vi "Manipulate outputs.vi"(1 "ON for":dbl, 4 "data value reference in":refnum<data-value>, 7 "Output pins":T1, 8 "Last on":timestamp, 9 "Delay":dbl, 10 "Threshold":dbl, 11 "Data":dbl) -> (0 "Time Output":timestamp, 2 "LED value":dbl, 3 "Fan value":dbl, 5 "data value reference out":refnum<data-value>)   [LabVIEW 2020]
uses:
  <vilib>/DAQmx/write.llb/DAQmx Write (Analog DBL 1Chan 1Samp).vi
  Global variable.vi
  <vilib>/DAQmx/miscellaneous.llb/DAQmx Fill In Error Info.vi
panel:
  in  "Decay speed":dbl=1.0
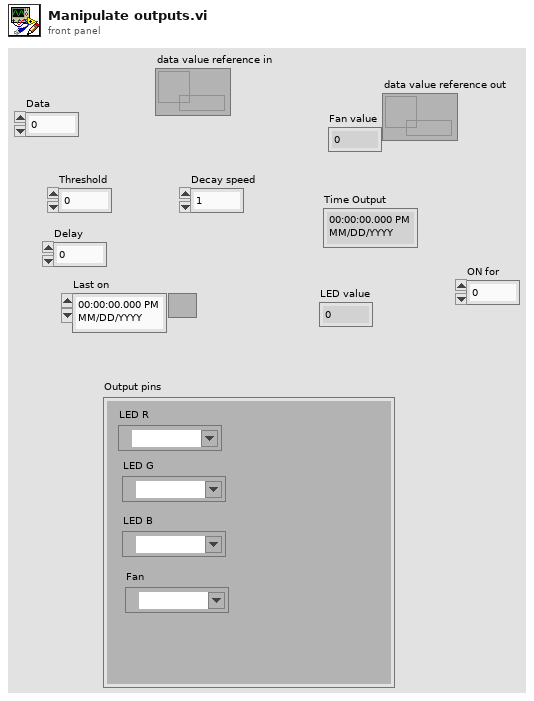
[diagram p1: front panel]
types:
  T1 = cluster{"LED R":tag, "LED G":tag, "LED B":tag, "Fan":tag}
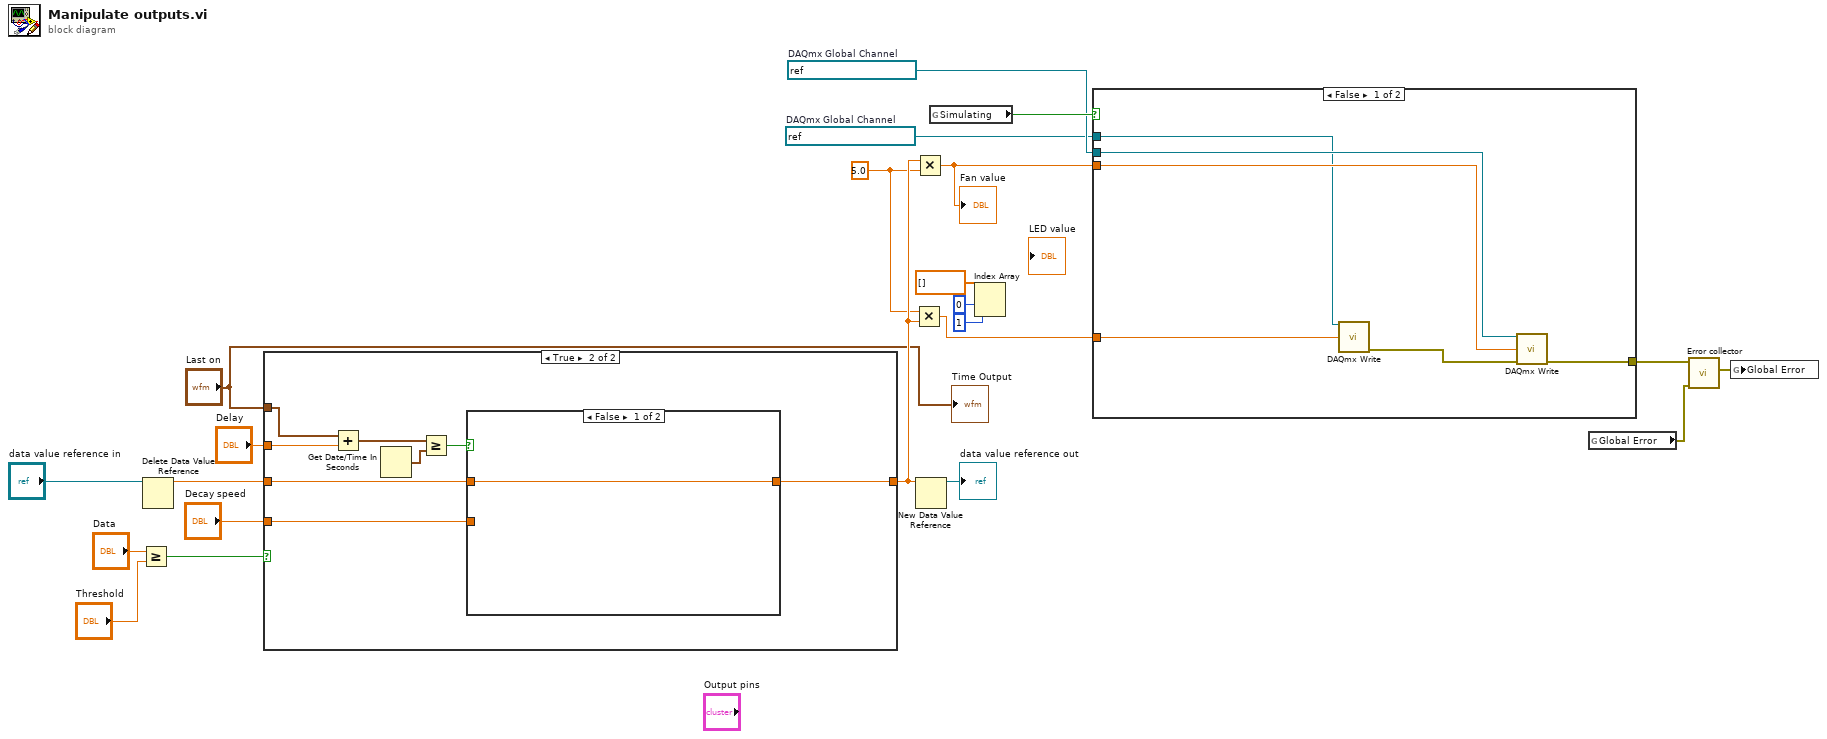
[diagram p0: block diagram]
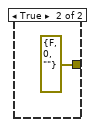
[diagram p2: hidden frame]
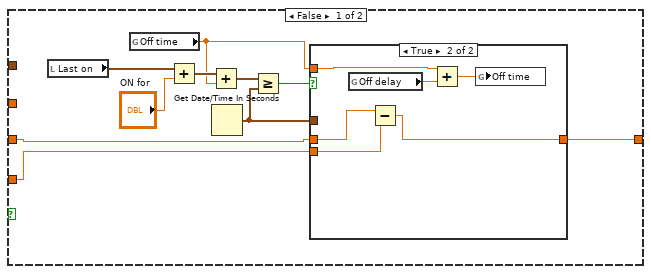
[diagram p3: hidden frame]
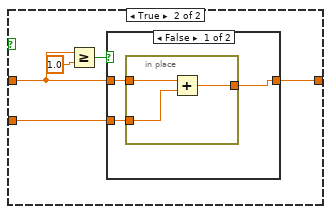
[diagram p5: hidden frame]
diagram:
  w6 = refnum<k21> "LEDOutputChannel"  # DAQmx Global Channel
  w7 = refnum<k21> "FanOutputChannel"  # DAQmx Global Channel
  w5 = 5.0
  n1 = Greater Or Equal?(x="Data", y="Threshold") -> (x >= y?=w20:bool)
  n2 = Delete Data Value Reference(data value reference="data value reference in") -> (data value=w16:dbl)  [unwired: 1 in, 1 out]
  n3 = case shown="True" w20 {
    tunnel: "Delay" -> [_ w47]
    tunnel: w16 -> [w28 w43]
    tunnel: "Decay speed" -> [w29 w42]
    tunnel: [w27 w41] -> w14
    tunnel: "Last on" -> [_ w40]
    frame False {
      n4 = local read "Last on"() -> (w31:timestamp)
      n5 = global read "Global variable.vi" "Off time"() -> (w23:dbl)
      n6 = Add(x=w31, y="ON for") -> (x+y=w24:timestamp)
      n7 = Add(x=w24, y=w23) -> (x+y=w25:timestamp)
      n8 = Get Date/Time In Seconds() -> (seconds since 1Jan1904=w26:timestamp)
      n9 = Greater Or Equal?(x=w25, y=w26) -> (x >= y?=w30:bool)
      n10 = case shown="True" w30 {
        tunnel: w29 -> [_ w39]
        tunnel: w28 -> [w33 w38]
        tunnel: [w33 w37] -> w27
        tunnel: w26 -> [_ _]
        tunnel: w23 -> [_ w35]
        frame False {
        }
        frame True {
          n11 = global read "Global variable.vi" "Off delay"() -> (w34:dbl)
          n12 = Subtract(x=w38, y=w39) -> (x-y=w37:dbl)
          n13 = Add(x=w35, y=w34) -> (x+y=w36:dbl)
          n14 = global write "Global variable.vi" "Off time"(w36) -> ()
        }
      }
    }
    frame True {
      n15 = Add(x=w40, y=w47) -> (x+y=w46:timestamp)
      n16 = Get Date/Time In Seconds() -> (seconds since 1Jan1904=w45:timestamp)
      n17 = Greater Or Equal?(x=w46, y=w45) -> (x >= y?=w44:bool)
      n18 = case shown="False" w44 {
        tunnel: w43 -> [w48 w51]
        tunnel: w42 -> [_ w50]
        tunnel: [w48 w49] -> w41
        frame False {
        }
        frame True {
          n19 = Greater Or Equal?(x=w51, y=1.0) -> (x >= y?=w52:bool)
          n20 = case shown="False" w52 {
            tunnel: w51 -> [w56 w60]
            tunnel: w50 -> [w55 _]
            tunnel: [w54 w60] -> w49
            frame False {
              n21 = in-place {
                in-place-border: w56 -> [w59]
                in-place-border: w55 -> [w58]
                in-place-border: [w57] -> w54
                n22 = Add(x=w59, y=w58) -> (x+y=w57:dbl)
              }
            }
            frame True {
            }
          }
        }
      }
    }
  }
  n23 = Multiply(x=w5, y=w14) -> (x*y=w2:dbl)
  n24 = Multiply(x=w14, y=w5) -> (x*y=w12:dbl)
  "Fan value" <- w12
  n25 = New Data Value Reference(data value=w14) -> (data value reference=→"data value reference out":refnum<data-value>)  [unwired: 1 in, 1 out]
  n26 = global read "Global variable.vi" "Simulating"() -> (w13:bool)
  n27 = Index Array(array=dbl[] [], index #1=0 ("index"), index #2=1 ("index")) -> ()  [unwired: 2 out]
  n28 = case shown="False" w13 {
    tunnel: w7 -> [w66 _]
    tunnel: w12 -> [w65 _]
    tunnel: [w64 errorcluster {"status"=FALSE, "code"=0, "source"=""} ("error out")] -> w9
    tunnel: w6 -> [w62 _]
    tunnel: w2 -> [w61 _]
    frame False {
      n29 = call-poly <vilib>:"DAQmx Write.vi"("task/channels in"=w62, "data"=w61) -> ("error out"=w63:errorcluster)  [unwired: 11 in, 2 out]
      n30 = call-poly <vilib>:"DAQmx Write.vi"("task/channels in"=w66, "data"=w65, "error in"=w63) -> ("error out"=w64:errorcluster)  [unwired: 10 in, 2 out]
    }
    frame True {
    }
  }
  n31 = global read "Global variable.vi" "Global Error"() -> (w11:errorcluster)
  n32 = call "Error collector.vi"("error list"=w11, "error in"=w9) -> ("error out"=w10:errorcluster)  [unwired: 9 in]
  n33 = global write "Global variable.vi" "Global Error"(w10) -> ()
  "Time Output" <- "Last on"
